vi "nirvififoEmulationGetNumberOfElementsToWrite.vi"(5 "Width":i32=1024, 7 "ErrorIn":bool, 8 "Name":string="simul", 9 "Local? (F)":bool, 14 "Size":i32=1024, 15 "ref in wired":bool, 16 "Type":variant, 17 "Update Size?":bool) -> (24 "Number of Elements to Write":u32)   [LabVIEW 2017]
uses:
  <instcachedir>/0/nirviFifoEmulationQueueMgr_E5CAEC123FF24DC58D834DCA3CDAA9B5.lvgen/nirviFifoEmulationQueueMgr_E5CAEC123FF24DC58D834DCA3CDAA9B5_000.vi
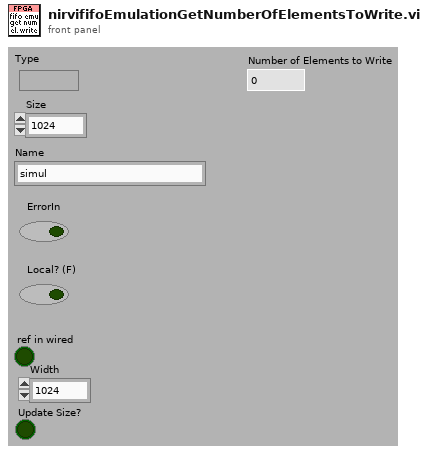
[diagram p1: front panel]
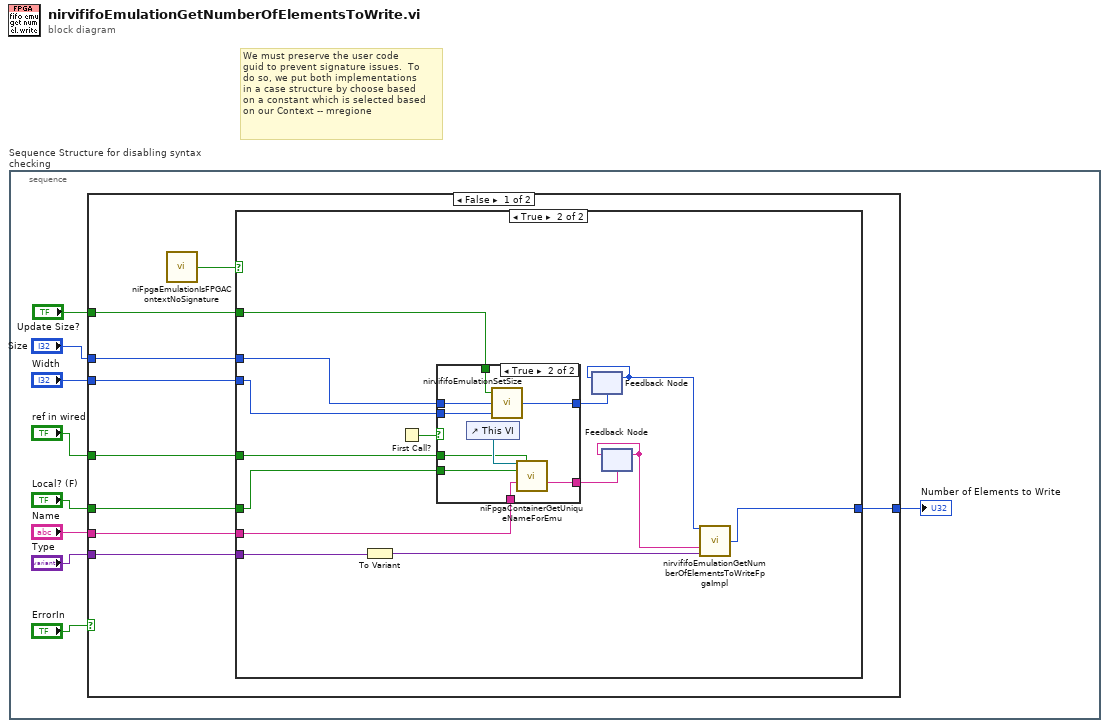
[diagram p0: block diagram]
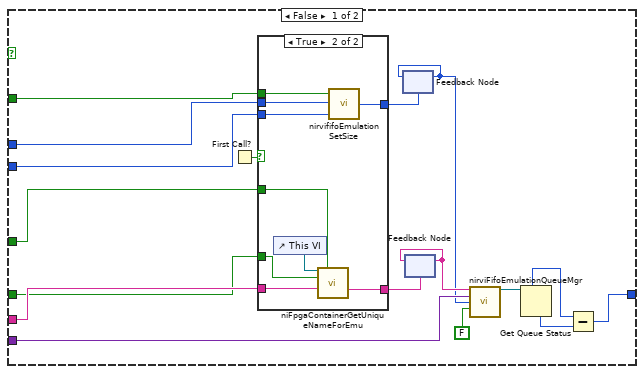
[diagram p2: hidden frame]
diagram:
  # "We must preserve the user code\nguid to prevent signature issues.  To\ndo so, we put both implementations\nin a case structure by choose based\non a constant which is selected based\non our Context -- mregione"
  n1 = stacked-sequence "Sequence Structure for disabling syntax checking" {
    frame #0 {
      n2 = case shown="False" "ErrorIn" {
        tunnel: "Name" -> [w17 _]
        tunnel: "ref in wired" -> [w15 _]
        tunnel: "Local? (F)" -> [w16 _]
        tunnel: "Size" -> [w14 _]
        tunnel: "Type" -> [w18 _]
        tunnel: [w13 _] -> w3
        tunnel: "Update Size?" -> [w12 _]
        tunnel: "Width" -> [w11 _]
        frame False {
          n3 = call <vilib>:"niFpgaEmulationIsFPGAContextNoSignature.vi"() -> ("Is Fpga Context?"=w10:bool)  [unwired: 15 in]
          n4 = case shown="True" w10 {
            tunnel: w18 -> [w23 w54]
            tunnel: w17 -> [w35 w45]
            tunnel: w16 -> [w34 w46]
            tunnel: w15 -> [w33 w47]
            tunnel: w14 -> [w32 w51]
            tunnel: [w19 w53] -> w13
            tunnel: w12 -> [w31 w52]
            tunnel: w11 -> [w30 w50]
            frame False {
              n5 = First Call?() -> (First Call?: T/F=w29:bool)
              n6 = case shown="True" w29 {
                tunnel: w35 -> [_ w41]
                tunnel: w32 -> [_ w44]
                tunnel: w34 -> [_ w39]
                tunnel: w33 -> [_ w38]
                tunnel: w31 -> [_ w43]
                tunnel: w30 -> [_ w42]
                tunnel: [_ w37] -> w25
                tunnel: [_ w36] -> w26
                frame False {
                }
                frame True {
                  n7 = control-ref of="This VI"() -> (w40:refnum<vi>)
                  n8 = call <vilib>:"niFpgaContainerGetUniqueNameForEmu.vi"("parent VI"=w40, "ref in wired"=w38, "local"=w39, "name in"=w41) -> ("name out"=w37:string)  [unwired: 11 in]
                  n9 = call <vilib>:"nirvififoEmulationSetSize.vi"("width"=w42, "Size"=w44, "Update?"=w43) -> ("Actual Size"=w36:i32)
                }
              }
              n10 = feedback #1(w26) -> (w22:i32)
              n11 = feedback-in #1(w22) -> ()
              n12 = feedback #2(w25) -> (w24:string)
              n13 = feedback-in #2(w24) -> ()
              n14 = call-generic <vilib>:"nirviFifoEmulationQueueMgr.vi"("FIFO Name"=w24, "Element"=w23, "Size"=w22, "Is Handshake?"=FALSE) -> ("FIFO"=w20:refnum<queue>)  [unwired: 11 in]
              n15 = Get Queue Status(queue=w20) -> (max queue size=w28:i32, # elements in queue=w27:i32)  [unwired: 2 in, 6 out]
              n16 = Subtract(x=w28, y=w27) -> (x-y=w19:u32)
            }
            frame True {
              n17 = To Variant(anything=w54) -> (Variant=w58:variant)
              n18 = First Call?() -> (First Call?: T/F=w57:bool)
              n19 = case shown="True" w57 {
                tunnel: [_ w66] -> w56
                tunnel: w52 -> [_ w65]
                tunnel: w51 -> [_ w64]
                tunnel: w50 -> [_ w63]
                tunnel: [_ w62] -> w49
                tunnel: w47 -> [_ w61]
                tunnel: w46 -> [_ w60]
                tunnel: w45 -> [_ w59]
                frame False {
                }
                frame True {
                  n20 = control-ref of="This VI"() -> (w67:refnum<vi>)
                  n21 = call <vilib>:"nirvififoEmulationSetSize.vi"("width"=w63, "Size"=w64, "Update?"=w65) -> ("Actual Size"=w62:i32)
                  n22 = call <vilib>:"niFpgaContainerGetUniqueNameForEmu.vi"("parent VI"=w67, "ref in wired"=w61, "local"=w60, "name in"=w59) -> ("name out"=w66:string)  [unwired: 11 in]
                }
              }
              n23 = feedback #3(w49) -> (w48:i32)
              n24 = feedback-in #3(w48) -> ()
              n25 = feedback #4(w56) -> (w55:string)
              n26 = feedback-in #4(w55) -> ()
              n27 = call <vilib>:"nirvififoEmulationGetNumberOfElementsToWriteFpgaImpl.vi"("Size"=w48, "Name"=w55, "Init Val"=w58) -> ("num to write"=w53:i64)  [unwired: 12 in]
            }
          }
        }
        frame True {
        }
      }
      "Number of Elements to Write" <- w3
    }
  }
